vi "PH_StatusHandler.set Status to color GUI Object for Color Blinds.vi"(1 "Ref CB State":refnum<vi>, 2 "Ref State":refnum<vi>, 3 "State":T1 caption="Enabling State" items=["no info", "off/false/out", "on/true/in", "Failure", "Alarm", "Status 1", "Status 2", "Status 3"], 4 "Blinking? (false)":bool, 5 "error in":errorcluster, 6 "Disabled? (false)":bool, 8 "Visible? (true)":bool=TRUE) -> (19 "error out":errorcluster)   [LabVIEW 2014, in "PH_StatusHandler.lvlib"]
doc: "This VI is forseen to indicate stati in PHELIX GUIs in order to support color blind persons. Besides the main color box (whichs reference must be connected to \"Ref State\"), an additional small color box must be connected to \"Ref CB State\". Both can be made visible (default: true), disabled (false), and blinking (false). The \"Enabling State\" has this effect:\n\nStatus Ref State Ref CB State Tip Strip\nno info (0) blue (0) gray (6) no information available \noff/false/out (1) darkgreen (1) darkgreen (1) off or false\non/true/in (2) lightgreen (2) lightgreen (2) on or true\nFailure (3) yellow (3) black (5) Failure \nAlarm (4) red (4) gray (6) Alarm \nStatus 1 (6) black (5) blue (0) Status 1\nStatus 2 (7) black (5) darkgreen (1) Status 2\nStatus 3 (8) black (5) lightgreen (2) Status 3"
uses:
  PH_StatusHandler.lvlib
  PH_StatusHandler.Status.ctl
  PH_Common/PH_Common.lvlib
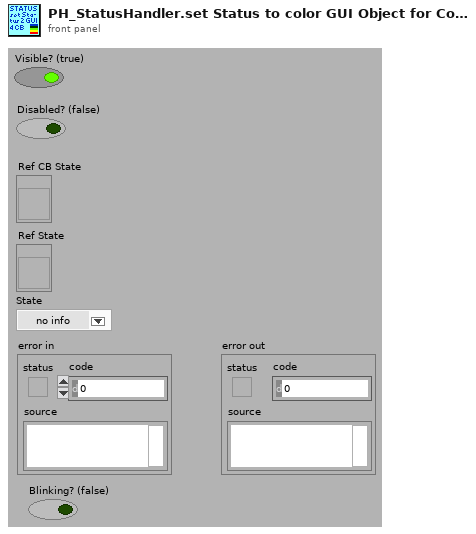
[diagram p1: front panel]
types:
  T1 = typedef "PH_StatusHandler.lvlib/PH_StatusHandler.Status.ctl" = i16
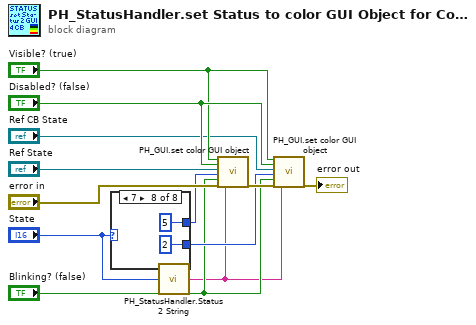
[diagram p0: block diagram]
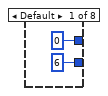
[diagram p2: hidden frame]
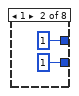
[diagram p3: hidden frame]
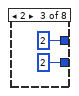
[diagram p4: hidden frame]
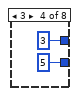
[diagram p5: hidden frame]
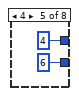
[diagram p6: hidden frame]
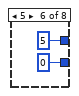
[diagram p7: hidden frame]
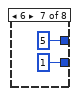
[diagram p8: hidden frame]
diagram:
  n1 = case shown="7" "State" {
    tunnel: [0 ("State") 1 ("State") 2 ("State") 3 ("State") 4 ("State") 5 ("State") 5 ("State") 5 ("State")] -> w4
    tunnel: [6 ("State") 1 ("State") 2 ("State") 5 ("State") 6 ("State") 0 ("State") 1 ("State") 2 ("State")] -> w10
    frame Default {
    }
    frame 1 {
    }
    frame 2 {
    }
    frame 3 {
    }
    frame 4 {
    }
    frame 5 {
    }
    frame 6 {
    }
    frame 7 {
    }
  }
  n2 = call "PH_StatusHandler.Status 2 String.vi"("Status"="State") -> ("Status as string"=w1:string)
  n3 = call "PH_GUI.set color GUI object.vi"("Visible? (true)"="Visible? (true)", "Disabled? (false)"="Disabled? (false)", "GUI object Ref"="Ref State", "State"=w4, "Blinking? (false)"="Blinking? (false)", "error in (no error)"="error in", "Tip Strip (N/A)"=w1) -> ("error out"=w12:errorcluster)  [unwired: 12 in]
  n4 = call "PH_GUI.set color GUI object.vi"("Visible? (true)"="Visible? (true)", "Disabled? (false)"="Disabled? (false)", "GUI object Ref"="Ref CB State", "State"=w10, "Blinking? (false)"="Blinking? (false)", "error in (no error)"=w12, "Tip Strip (N/A)"=w1) -> ("error out"=→"error out":errorcluster)  [unwired: 12 in]
